vi "DIO Readback.vi"(7 "Box ID":u8=1, 8 "error in (no error)":errorcluster, 11 "CAN in":refnum<class "XNET_BS120x.lvclass">) -> (0 "error out":errorcluster, 2 "DIO Readback":bool[](array[boolean]), 3 "CAN out":refnum<class "XNET_BS120x.lvclass">)   [LabVIEW 2021, in "BS120x Driver.lvlib" / "XNET_BS120x.lvclass"]
uses:
  XNET_BS120x.lvclass
  BS120x.lvclass
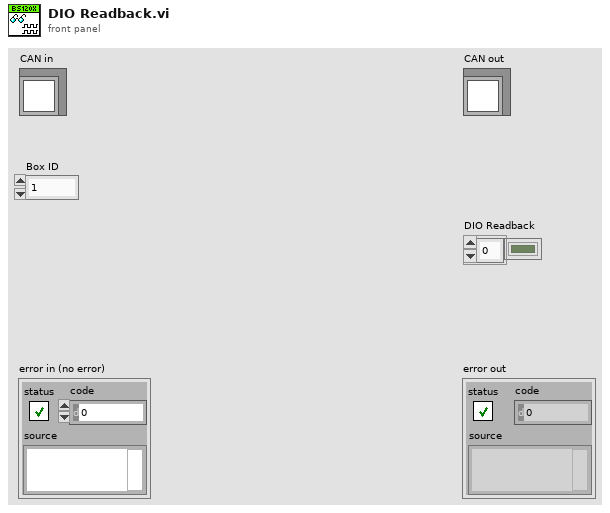
[diagram p1: front panel]
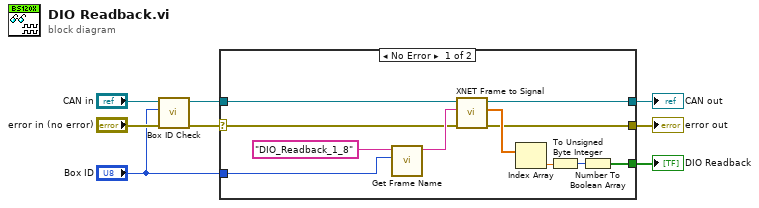
[diagram p0: block diagram]
diagram:
  n1 = call "Box ID Check.vi"("error in (no error)"="error in (no error)", "Box ID"="Box ID", "CAN in"="CAN in") -> ("error out"=w3:errorcluster, "CAN out"=w4:refnum<class "XNET_BS120x.lvclass">)  [unwired: 7 in]
  n2 = case shown="No Error" w3 {
    selector: w3 -> [w9 w20]
    tunnel: [w17 _] -> w8
    tunnel: w4 -> [w16 w21]
    tunnel: [w14 w20] -> w6
    tunnel: [w13 w21] -> w5
    tunnel: "Box ID" -> [w10 _]
    frame No Error {
      n3 = call "Get Frame Name.vi"("Box ID"=w10, "Frame Name"="DIO_Readback_1_8" ("Frame")) -> ("Frame Name out"=w11:string)  [unwired: 9 in]
      n4 = call "XNET Frame to Signal.vi"("error in (no error)"=w9, "Frame"=w11, "CAN in"=w16) -> ("error out"=w14:errorcluster, "signal data"=w15:dbl[], "CAN out"=w13:refnum<class "XNET_BS120x.lvclass">)  [unwired: 6 in]
      n5 = Index Array(array=w15) -> (element=w19:dbl)  [unwired: 1 in]
      n6 = To Unsigned Byte Integer(number=w19) -> (unsigned 8bit integer=w18:u8)
      n7 = Number To Boolean Array(number=w18) -> (Boolean array=w17:bool[])
    }
    frame Error {
    }
  }
  "error out" <- w6
  "CAN out" <- w5
  "DIO Readback" <- w8
